vi "MAIN_TL_define_parameters.vi"(5 "queue DAQ":refnum<queue>, 7 "TL - setpoint cluster":T2, 8 "error in":errorcluster, 9 "variant":variant, 10 "Start acquisition":bool, 11 "TL - Laser cluster":T1={"405"=0.0, "488"=0.0, "561"=0.0, "641"=0.0, "BF "=0.0, "405 setpoint"=FALSE, "488 setpoint"=FALSE, "561 setpoint"=FALSE, "641 setpoint"=FALSE, "BF setpoint"=FALSE, "N planes 405"=0, "Dz 405"=0, "N planes 488"=0, "Dz 488"=0, "N planes 561"=0, "Dz 561"=0, "N planes 641"=0, "Dz 641"=0, "N planes BF"=0, "Dz BF"=0, "Tau 405"=inf, "Tau 488"=inf, "Tau 561"=inf, "Tau 641"=inf, "Tau BF"=inf, "405 set"=FALSE, "488 set "=FALSE, "561 set"=FALSE, "641 set"=FALSE, "BF set"=FALSE} {"Tau BF" format="%#_6e"; "Tau 641" format="%#_6e"; "Tau 561" format="%#_6e"; "Tau 488" format="%#_6e"; "Tau 405" format="%#_6e"; "641" min=0.0 max=100.0 step=0.1 scale=0.0..100.0; "561" min=0.0 max=100.0 step=0.1 scale=0.0..100.0; "405" min=0.0 max=100.0 step=0.1 scale=0.0..100.0; "488" min=0.0 max=100.0 step=0.1 scale=0.0..100.0; "BF" min=0.0 max=100.0 step=0.1 scale=0.0..100.0}) -> (0 "error out":errorcluster, 2 "Next task":T3, 3 "TL - setpoint cluster OUT":T2, 4 "TL - Laser cluster OUT":T1={"405"=0.0, "488"=0.0, "561"=0.0, "641"=0.0, "BF "=0.0, "405 setpoint"=FALSE, "488 setpoint"=FALSE, "561 setpoint"=FALSE, "641 setpoint"=FALSE, "BF setpoint"=FALSE, "N planes 405"=0, "Dz 405"=0, "N planes 488"=0, "Dz 488"=0, "N planes 561"=0, "Dz 561"=0, "N planes 641"=0, "Dz 641"=0, "N planes BF"=0, "Dz BF"=0, "Tau 405"=inf, "Tau 488"=inf, "Tau 561"=inf, "Tau 641"=inf, "Tau BF"=inf, "405 set"=FALSE, "488 set "=FALSE, "561 set"=FALSE, "641 set"=FALSE, "BF set"=FALSE} {"Tau BF" format="%#_6e"; "Tau 641" format="%#_6e"; "Tau 561" format="%#_6e"; "Tau 488" format="%#_6e"; "Tau 405" format="%#_6e"; "641" min=0.0 max=100.0 step=0.1 scale=0.0..100.0; "561" min=0.0 max=100.0 step=0.1 scale=0.0..100.0; "405" min=0.0 max=100.0 step=0.1 scale=0.0..100.0; "488" min=0.0 max=100.0 step=0.1 scale=0.0..100.0; "BF" min=0.0 max=100.0 step=0.1 scale=0.0..100.0})   [LabVIEW 2015]
uses:
  CONTROLS/Q_main_element.ctl
  CONTROLS/Q_DAQ_element.ctl
  CONTROLS/Time_lapse_parameters.ctl
  GLOBAL/Global_DAQ.vi
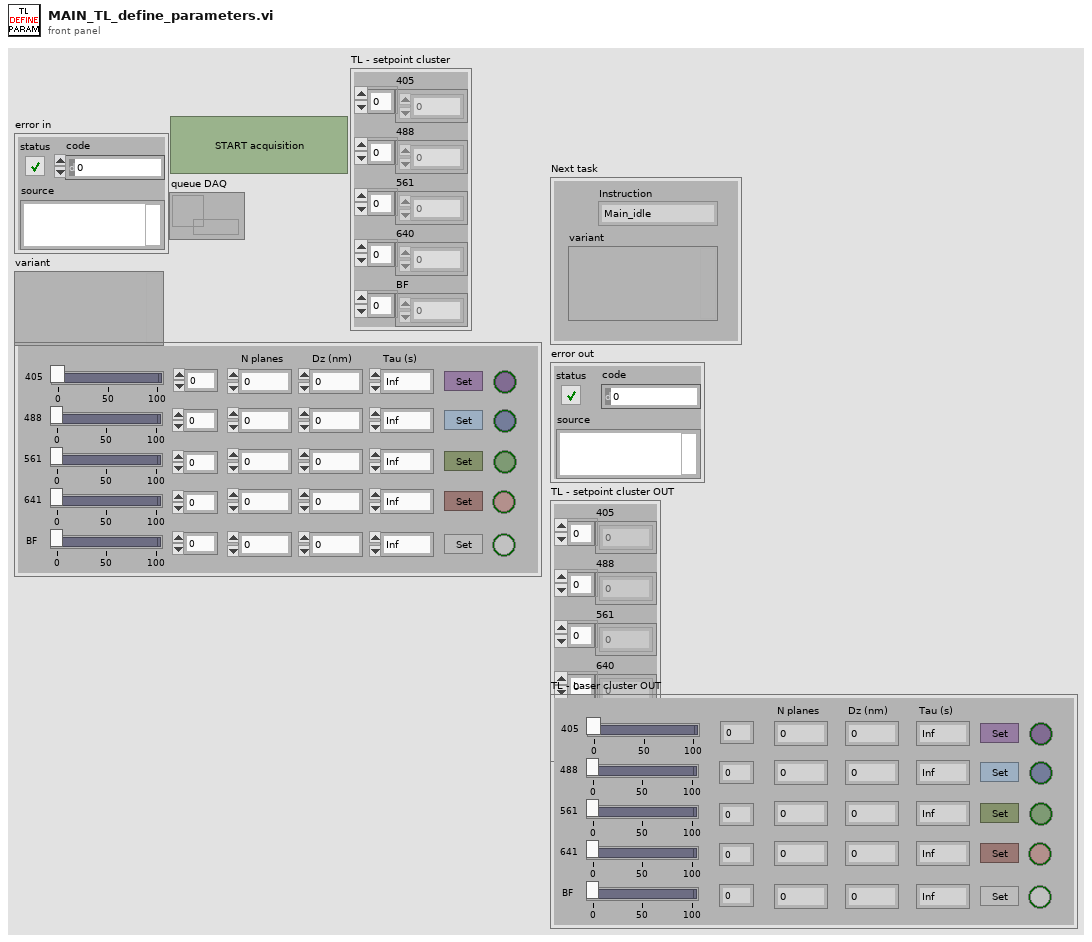
[diagram p1: front panel]
types:
  T1 = typedef "Time_lapse_parameters.ctl" = cluster{"405":dbl, "488":dbl, "561":dbl, "641":dbl, "BF ":dbl, "405 setpoint":bool, "488 setpoint":bool, "561 setpoint":bool, "641 setpoint":bool, "BF setpoint":bool, "N planes 405":i32, "Dz 405":i32, "N planes 488":i32, "Dz 488":i32, "N planes 561":i32, "Dz 561":i32, "N planes 641":i32, "Dz 641":i32, "N planes BF":i32, "Dz BF":i32, "Tau 405":dbl, "Tau 488":dbl, "Tau 561":dbl, "Tau 641":dbl, "Tau BF":dbl, "405 set":bool, "488 set ":bool, "561 set":bool, "641 set":bool, "BF set":bool}
  T2 = cluster{"405":dbl[], "488":dbl[], "561":dbl[], "640":dbl[], "BF":dbl[]}
  T3 = typedef "Q_main_element.ctl" = cluster{"variant":variant, "Instruction":enum16{"Main_idle", "Main_initialize", "Main_initialize_TDMS", "Main_initialize_Queue", "Main_error", "Main_DAQ_initialization_results", "Main_ASI_initialization_results", "Main_Piezo_initialization_results", "Main_Valve_initialization_results", "Main_Pump_initialization_results", "Main_CAMERA_initialization_results", "Main_DAQ_error", "Main_ASI_error", "Main_Piezo_error", "Main_CAMERA_error", "Main_Valve_error", "Main_Pump_error", "Main_start_acquiring", "Main_not_acquiring", "Main_acquiring", "Main_stop_acquiring", "Main_change_exposure", "Main_change_z_scan_parameters", "Main_define_ROI", "Main_define_mosaic", "Main_read_kinetic_time", "Main_cooler", "Main_read_temperature", "Main_save_XY", "Main_load_XY", "Main_discard_XY", "Main_move_to_XY", "Main_measure_QPD", "Main_autofocus_calibration", "Main_save_PID", "Main_change_H_valve_position", "Main_two_way_valve", "Main_save_movie", "Main_init_single_scan", "Main_single_scan", "Main_stop_single_scan", "Main_merFISH_illumination_parameters", "Main_merFISH_buffer_probe_list", "Main_merFISH_injections_procedure", "Main_merFISH_save_setpoint", "Main_merFISH_DAPI_parameters", "Main_merFISH_Brightfield_parameters", "Main_merFISH_save_embryo_ROI", "Main_merFISH_init", "Main_merFISH_resume", "Main_merFISH_start_autofocus", "Main_merFISH_open_close_valve_merFISH", "Main_merFISH_open_close_valve_photobleaching", "Main_merFISH_hybridization", "Main_merFISH_move_to_ROI", "Main_merFISH_wait_stabilization", "Main_merFISH_scan_laser", "Main_merFISH_scan_brightfield", "Main_merFISH_photobleaching_injection", "Main_merFISH_photobleaching", "Main_merFISH_save", "Main_merFISH_send_email", "Main_merFISH_close", "Main_TL_define_parameters", "Main_TL_reset_parameters", "Main_TL_init", "Main_TL_start_autofocus", "Main_TL_move_to_ROI", "Main_TL_wait_for_stabilization", "Main_TL_scan", "Main_TL_wait_cycle_end", "Main_TL_close", "Main_STOP"}}
  T4 = typedef "Q_DAQ_element.ctl" = cluster{"variant":variant, "Instruction":enum16{"DAQ_idle", "DAQ_initialize", "DAQ_error", "DAQ_security_stop", "DAQ_start_QPD", "DAQ_change_QPD_display", "DAQ_read_display_QPD_signal", "DAQ_QPD_init_autofocus", "DAQ_read_display_send_QPD_signal", "DAQ_close_autofocus_calibration_ramp", "DAQ_close_autofocus", "DAQ_405", "DAQ_488", "DAQ_561", "DAQ_641", "DAQ_zero_all", "DAQ_init_single_scan", "DAQ_single_scan", "DAQ_two_way_valve", "DAQ_init_merFISH", "DAQ_scan_merFISH", "DAQ_photobleaching_merFISH", "DAQ_close_merFISH", "DAQ_init_TL", "DAQ_synchro_TL", "DAQ_close_task_TL", "DAQ_close_TL", "DAQ_stop"}}
  T5 = enum16{"DAQ_idle", "DAQ_initialize", "DAQ_error", "DAQ_security_stop", "DAQ_start_QPD", "DAQ_change_QPD_display", "DAQ_read_display_QPD_signal", "DAQ_QPD_init_autofocus", "DAQ_read_display_send_QPD_signal", "DAQ_close_autofocus_calibration_ramp", "DAQ_close_autofocus", "DAQ_405", "DAQ_488", "DAQ_561", "DAQ_641", "DAQ_zero_all", "DAQ_init_single_scan", "DAQ_single_scan", "DAQ_two_way_valve", "DAQ_init_merFISH", "DAQ_scan_merFISH", "DAQ_photobleaching_merFISH", "DAQ_close_merFISH", "DAQ_init_TL", "DAQ_synchro_TL", "DAQ_close_task_TL", "DAQ_close_TL", "DAQ_stop"}
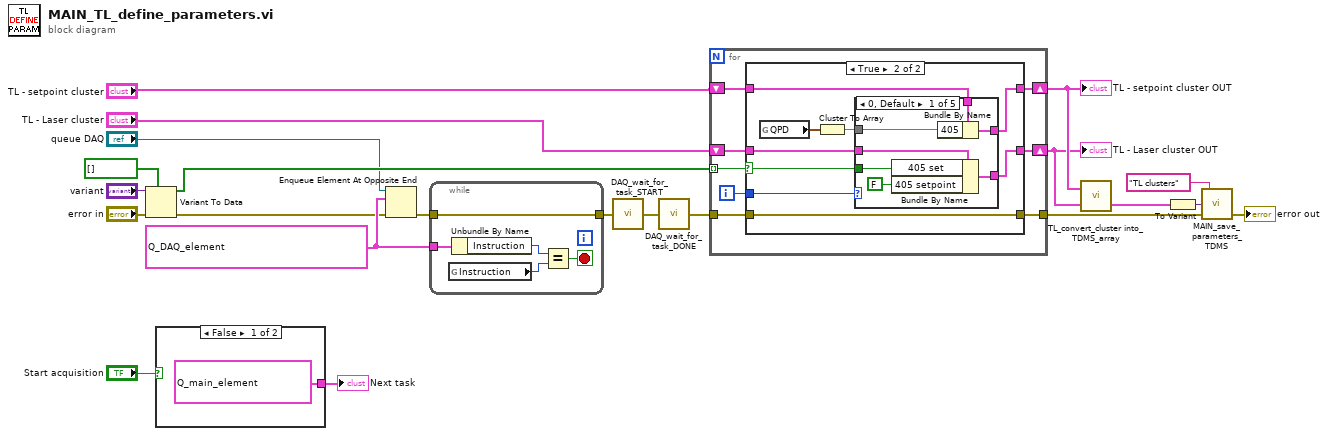
[diagram p0: block diagram]
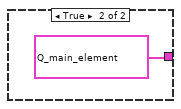
[diagram p2: hidden frame]
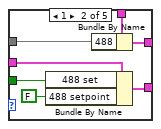
[diagram p4: hidden frame]
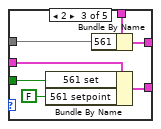
[diagram p5: hidden frame]
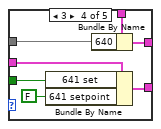
[diagram p6: hidden frame]
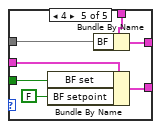
[diagram p7: hidden frame]
diagram:
  w22 = T4 {"variant"=variant, "Instruction"=enum."DAQ_read_display_send_QPD_signal"} ("element")
  n1 = Variant To Data(error in="error in", type=bool[] [] ("array"), Variant="variant") -> (data=w12:bool[], error out=w10:errorcluster)
  n2 = case shown="False" "Start acquisition" {
    tunnel: [T3 {"variant"=variant, "Instruction"=enum."Main_not_acquiring"} ("Q_main_element") T3 {"variant"=variant, "Instruction"=enum."Main_acquiring"} ("Q_main_element")] -> w5
    frame False {
    }
    frame True {
    }
  }
  "Next task" <- w5
  n3 = Enqueue Element At Opposite End(queue="queue DAQ", element=w22, error in (no error)=w10) -> (error out=w20:errorcluster)  [unwired: 1 in, 2 out]
  n4 = while {
    tunnel: w20 -> [w26]
    tunnel: [w26] -> w21
    tunnel: w22 -> [w25]
    stop <- w28 stop-if-true
    n5 = global read "Global_DAQ.vi" "Instruction"() -> (w29:T5)
    n6 = Unbundle By Name(w25) -> ("Instruction"=w27:T5)
    n7 = Equal?(x=w27, y=w29) -> (x = y?=w28:bool)
  }
  n8 = call "DAQ_wait_for_task_START.vi"("error in"=w21) -> ("error out"=w9:errorcluster)
  n9 = call "DAQ_wait_for_task_DONE.vi"("error in"=w9) -> ("error out"=w13:errorcluster)
  n10 = for {
    tunnel: w12 -> [w37] mode=indexing
    tunnel: w13 -> [w34]
    tunnel: [w35] -> w16
    shift-right: [w32] -> w18
    shift-left: "TL - setpoint cluster" -> [w33]
    shift-right: [w30] -> w17
    shift-left: "TL - Laser cluster" -> [w31]
    i -> [w36]
    n11 = case shown="True" w37 {
      selector: w37 -> [_ w42]
      tunnel: w36 -> [_ w49]
      tunnel: [w40 w48] -> w35
      tunnel: w34 -> [w40 w48]
      tunnel: w33 -> [w39 w45]
      tunnel: [w39 w44] -> w32
      tunnel: w31 -> [w38 w43]
      tunnel: [w38 w41] -> w30
      frame False {
      }
      frame True {
        n12 = global read "Global_DAQ.vi" "QPD"() -> (w47:cluster{"X":dbl, "Y":dbl, "intensity":dbl})
        n13 = Cluster To Array(cluster=w47) -> (array=w46:dbl[])
        n14 = case shown="0, Default" w49 {
          tunnel: [w54 w61 w68 w75 w82] -> w44
          tunnel: w46 -> [w56 w63 w70 w77 w84]
          tunnel: w45 -> [w55 w62 w69 w76 w83]
          tunnel: w43 -> [w53 w60 w67 w74 w81]
          tunnel: w42 -> [w52 w59 w66 w73 w80]
          tunnel: [w51 w58 w65 w72 w79] -> w41
          frame 0, Default {
            n15 = Bundle By Name(cluster=w53, "405 set"=w52, "405 setpoint"=FALSE) -> (w51:T1)
            n16 = Bundle By Name(cluster=w55, "405"=w56) -> (w54:T2)
          }
          frame 1 {
            n17 = Bundle By Name(cluster=w60, "488 set"=w59, "488 setpoint"=FALSE ("405 setpoint")) -> (w58:T1)
            n18 = Bundle By Name(cluster=w62, "488"=w63) -> (w61:T2)
          }
          frame 2 {
            n19 = Bundle By Name(cluster=w67, "561 set"=w66, "561 setpoint"=FALSE ("405 setpoint")) -> (w65:T1)
            n20 = Bundle By Name(cluster=w69, "561"=w70) -> (w68:T2)
          }
          frame 3 {
            n21 = Bundle By Name(cluster=w74, "641 set"=w73, "641 setpoint"=FALSE ("405 setpoint")) -> (w72:T1)
            n22 = Bundle By Name(cluster=w76, "640"=w77) -> (w75:T2)
          }
          frame 4 {
            n23 = Bundle By Name(cluster=w81, "BF set"=w80, "BF setpoint"=FALSE ("405 setpoint")) -> (w79:T1)
            n24 = Bundle By Name(cluster=w83, "BF"=w84) -> (w82:T2)
          }
        }
      }
    }
  }
  "TL - setpoint cluster OUT" <- w18
  "TL - Laser cluster OUT" <- w17
  n25 = call "TL_convert_cluster into_TDMS_array.vi"("TL cluster"=w17, "TL - setpoint cluster"=w18) -> ("TL data for TDMS"=w19:cluster{dbl[][], dbl[][]})  [unwired: 1 in]
  n26 = To Variant(anything=w19) -> (Variant=w15:variant)
  n27 = call "MAIN_save_parameters_TDMS.vi"("error in"=w16, "Data"=w15, "Channel name"="TL clusters" ("group name")) -> ("error out"=→"error out":errorcluster)  [unwired: 2 in]
